vi "OTA Blink LED.vi"(8 "Error In":errorcluster) -> (0 "Error Out":errorcluster)   [LabVIEW 2014, in "ESP8266 WiFi Wrapper.lvlib"]
uses:
  ESP8266 WiFi Wrapper.lvlib
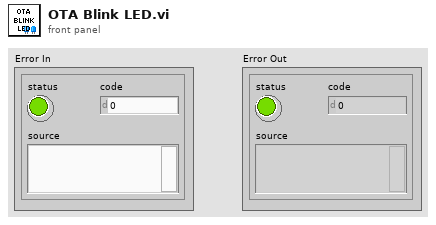
[diagram p1: front panel]
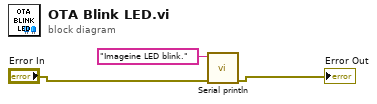
[diagram p0: block diagram]
diagram:
  n1 = call <vilib>:"Serial println.vi"("Error In"="Error In", "string in"="Imageine LED blink.") -> ("Error Out"=→"Error Out":errorcluster)  [unwired: 9 in]
